vi "Get Click Zone by Index.vi"(10 "index":i32, 11 "array in":T2) -> (1 "found?":bool, 2 "click zone":T1={"wheel index"=-1, "global coordinate"={"x"=0.0, "y"=0.0}, "radius"=0.0}, 3 "array out":T2)   [LabVIEW 2017, in "NI_Robotics_Configure Steering Frame.lvlib"]
uses:
  <vilib>/robotics/Dialog/Configure Steering Frame/NI_Robotics_Configure Steering Frame.lvlib
  <vilib>/robotics/Dialog/Configure Steering Frame/Click Zone.ctl
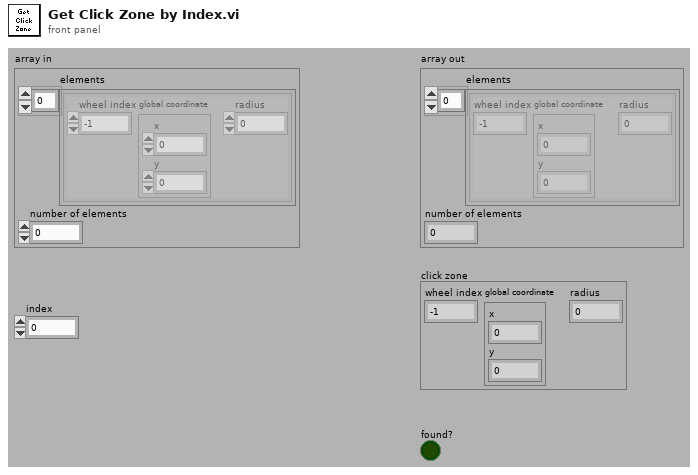
[diagram p1: front panel]
types:
  T1 = typedef "NI_Robotics_Configure Steering Frame.lvlib/Click Zone.ctl" = cluster{"wheel index":i32, "global coordinate":cluster{"x":dbl, "y":dbl}, "radius":dbl}
  T2 = cluster{"elements":T1[], "number of elements":i32}
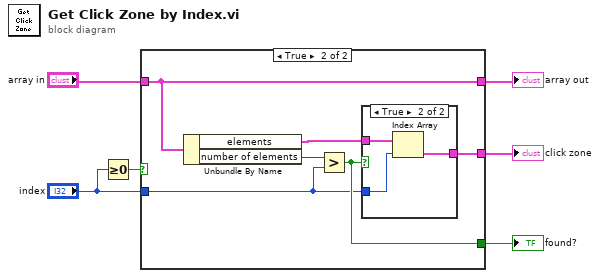
[diagram p0: block diagram]
diagram:
  n1 = Greater Or Equal To 0?(x="index") -> (x >= 0?=w6:bool)
  n2 = case shown="True" w6 {
    tunnel: [_ w12] -> w1
    tunnel: "array in" -> [w7 w8]
    tunnel: [_ w10] -> w2
    tunnel: "index" -> [_ w9]
    tunnel: [w7 w8] -> w3
    frame False {
    }
    frame True {
      n3 = Unbundle By Name(w8) -> ("elements"=w13:T1[], "number of elements"=w11:i32)
      n4 = Greater?(x=w11, y=w9) -> (0:w12:bool)
      n5 = case shown="True" w12 {
        tunnel: w13 -> [_ w16]
        tunnel: w9 -> [_ w15]
        tunnel: [_ w14] -> w10
        frame False {
        }
        frame True {
          n6 = Index Array(array=w16, index=w15) -> (element=w14:T1)
        }
      }
    }
  }
  "array out" <- w3
  "click zone" <- w2
  "found?" <- w1
